vi "Get Window RECT_KT.vi"(11 "hWnd":u32) -> (2 "RECT":T1, 3 "hWnd dup":u32)   [LabVIEW 2017, in "KTools.lvlib"]
doc: "<------Get Window Boundaries-------->\nReturns handle window boundaries"
uses:
  KTools.lvlib
  user32.dll
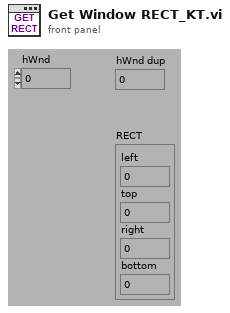
[diagram p1: front panel]
types:
  T1 = cluster{"left":i32, "top":i32, "right":i32, "bottom":i32}
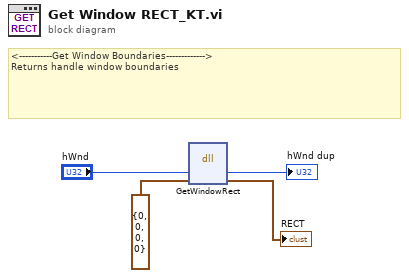
[diagram p0: block diagram]
diagram:
  # "<-----------Get Window Boundaries------------->\nReturns handle window boundaries"
  n1 = dll-call lib="user32.dll" fn="GetWindowRect"("hWnd"="hWnd", "RECT"=T1 {"left"=0, "top"=0, "right"=0, "bottom"=0}) -> ("hWnd"=→"hWnd dup":u32, "RECT"=→"RECT":T1)  [unwired: 4 in, 2 out]
